vi "configuration to node.vi"(8 "error in":errorcluster, 10 "CEF_Configuration":refnum<class "CEF_serializable configuration.lvclass">, 11 "CEF_Hierarchy repo in":refnum<class "CEF_HierarchyRepo.lvclass">) -> (0 "error out":errorcluster, 2 "CEF_Serialize node":refnum<class "CEF_serializable node.lvclass">, 3 "CEF_Hierarchy repo out":refnum<class "CEF_HierarchyRepo.lvclass">)   [LabVIEW 2023, in "CEF.lvlib" / "CEF_HierarchyRepo.lvclass"]
doc: "Copyright 2017 National Instruments Corporation\n\nLicensed under the Apache License, Version 2.0 (the \"License\"); you may not use this file except in compliance with the License. You may obtain a copy of the License at http://www.apache.org/licenses/LICENSE-2.0\nUnless required by applicable law or agreed to in writing, software distributed under the License is distributed on an \"AS IS\" BASIS, WITHOUT WARRANTIES OR CONDITIONS OF ANY KIND, either express or implied. See the License for the specific language governing permissions and limitations under the License."
uses:
  CEF_HierarchyRepo.lvclass
  serializable configuration/CEF_serializable configuration.lvclass
  serializable node/CEF_serializable node.lvclass
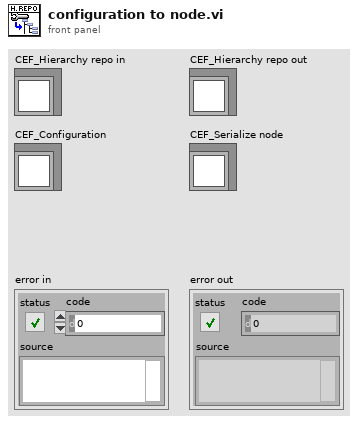
[diagram p1: front panel]
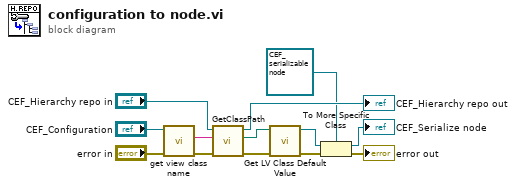
[diagram p0: block diagram]
diagram:
  n1 = call "get view class name.vi"("error in"="error in", "CEF_Configuration in"="CEF_Configuration") -> ("error out"=w9:errorcluster, "view class"=w8:string)  [unwired: 7 in, 1 out]
  n2 = call-dynamic "GetClassPath.vi"("error in"=w9, "class name"=w8, "CEF_Repository in"="CEF_Hierarchy repo in") -> ("error out"=w6:errorcluster, "class path"=w7:path, "CEF_Repository out"=→"CEF_Hierarchy repo out":refnum<class "CEF_HierarchyRepo.lvclass">)  [unwired: 6 in]
  n3 = call <vilib>:"Get LV Class Default Value.vi"("error in (no error)"=w6, "class path"=w7) -> ("error out"=w5:errorcluster, "object"=w4:refnum<class>)  [unwired: 8 in]
  n4 = To More Specific Class(target class=refnum<class "CEF_serializable node.lvclass"> refnum ("node"), reference=w4, error in=w5) -> (specific class reference=→"CEF_Serialize node":refnum<class "CEF_serializable node.lvclass">, error out=→"error out":errorcluster)
